vi "wavelength spectrum to time spectrum.vi"(9 "Zero padding":cluster{"zero pad":bool, "# Zeros":i32}={"zero pad"=FALSE, "# Zeros"=10000}, 10 "Input spectrum (nm)":T2, 11 "# interpolated points / # original points":i32=1) -> (1 "FFT of input spectrum":T1(graph) caption="Lineout graph", 2 "dt (s)":dbl, 3 "interpix spacing after interpolation (Hz)":dbl, 5 "Spectrum interpolated to even grid in frequency":T3(graph) caption="Lineout graph")   [LabVIEW 2013]
uses:
  <vilib>/Analysis/1siggen.llb/Ramp Pattern by Samples.vi
  <vilib>/Analysis/NI_AALPro.lvlib
  <vilib>/gmath/NI_Gmath.lvlib
  <vilib>/Analysis/NI_AALBase.lvlib
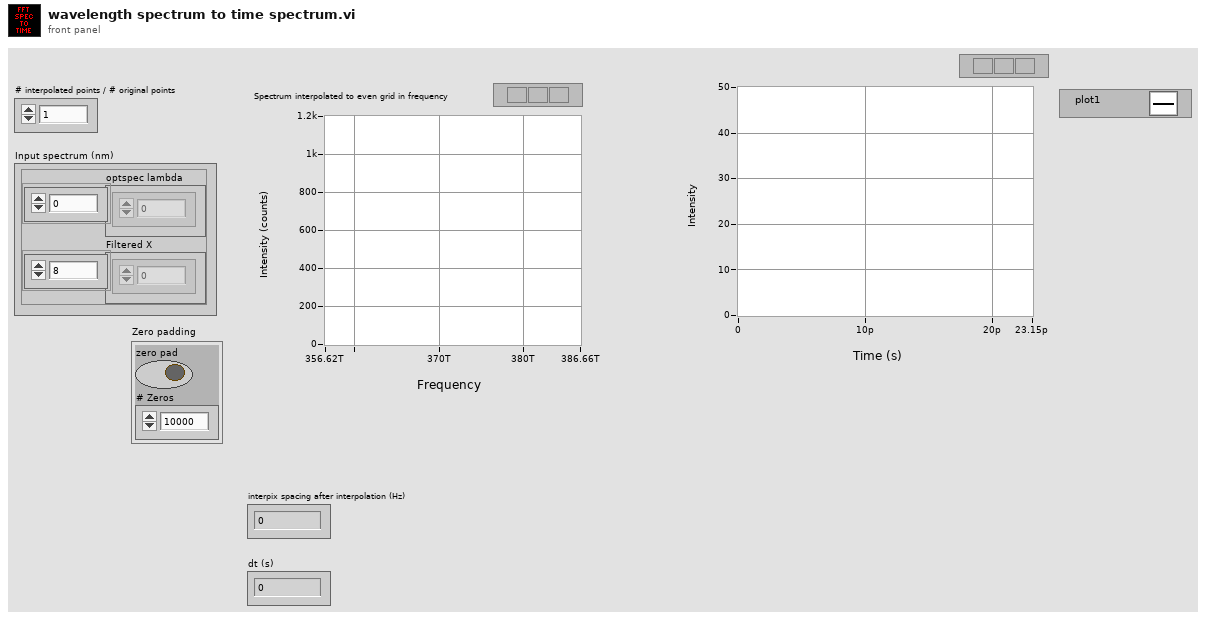
[diagram p1: front panel]
types:
  T1 = cluster{"Ramp Pattern":dbl[], "Amp Spectrum Mag (Vrms)":dbl[]}
  T2 = cluster{"optspec lambda":dbl[], "Filtered X":dbl[]}
  T3 = cluster{"optspec lambda":dbl[], "Filtered X":dbl[]}[]
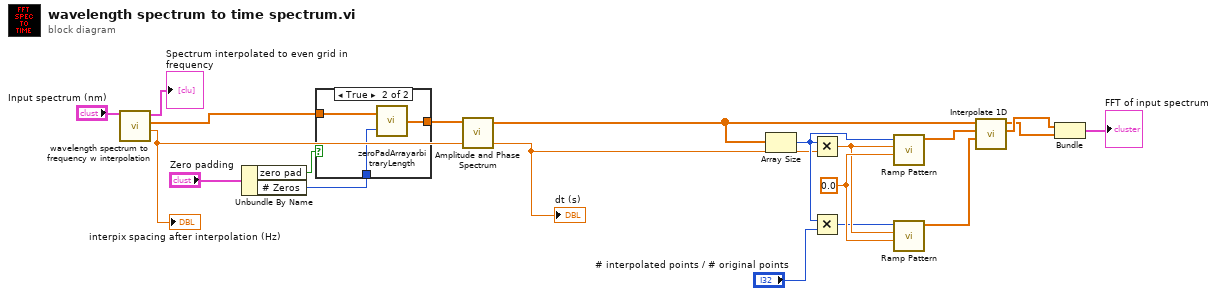
[diagram p0: block diagram]
diagram:
  w19 = 0.0 ("start")
  n1 = call "wavelength spectrum to frequency w interpolation.vi"("Input spectrum (nm)"="Input spectrum (nm)") -> ("interpix spacing after interpolation (Hz)"=w12:dbl, "interpolated amplitudes"=w5:dbl[], "spectrum and interpolated spectrum"=→"Spectrum interpolated to even grid in frequency":cluster{"Ramp Pattern":dbl[], "yi":dbl[]}[])  [unwired: 8 in]
  "interpix spacing after interpolation (Hz)" <- w12
  n2 = Unbundle By Name("Zero padding") -> ("zero pad"=w2:bool, "# Zeros"=w1:i32)
  n3 = case shown="True" w2 {
    tunnel: w5 -> [w21 w24]
    tunnel: [w21 w23] -> w4
    tunnel: w1 -> [_ w22]
    frame False {
    }
    frame True {
      n4 = call "zeroPadArrayarbitraryLength.vi"("# Zeros"=w22, "Array to Pad"=w24) -> ("Output Array"=w23:dbl[])
    }
  }
  n5 = call <vilib>:"Amplitude and Phase Spectrum.vi"("dt"=w12, "Signal (V)"=w4) -> ("df"=w11:dbl, "Amp Spectrum Mag (Vrms)"=w16:dbl[])  [unwired: 1 in, 1 out]
  "dt (s)" <- w11
  n6 = Array Size(array=w16) -> (size(s)=w14:i32)
  n7 = Multiply(x=w14, y=w11) -> (x*y=w18:dbl)
  n8 = Multiply(x=w14, y="# interpolated points / # original points") -> (x*y=w17:i32)
  n9 = call-poly <vilib>:"Ramp Pattern.vi"("start"=w19, "end"=w18, "samples"=w14) -> ("Ramp Pattern"=w15:dbl[])  [unwired: 7 in, 1 out]
  n10 = call-poly <vilib>:"Ramp Pattern.vi"("start"=w19, "end"=w18, "samples"=w17) -> ("Ramp Pattern"=w20:dbl[])  [unwired: 7 in, 1 out]
  n11 = call <vilib>:"Interpolate 1D.vi"("xi"=w20, "X"=w15, "Y"=w16) -> ("xi used"=w8:dbl[], "yi"=w7:dbl[])  [unwired: 6 in, 1 out]
  n12 = Bundle("xi used"=w8, "yi"=w7) -> (→"FFT of input spectrum":cluster{"xi used":dbl[], "yi":dbl[]})  [unwired: 1 in]
